vi "SetFlowRate.vi"(7 "Timeout (ms)":u32=2000, 8 "Error In":errorcluster, 10 "Flow Rate (mL/min)":dbl format="%.1f", 11 "Sierra M100 In":refnum<visa-resource-name>) -> (0 "Error Out":errorcluster, 2 "Set?":bool, 3 "Sierra M100 Out":refnum<visa-resource-name>)   [LabVIEW 2012, in "Sierra-M100.lvlib"]
doc: "This VI is sets the flow rate. Use this VI when unsure which of the other VIs to use for setting the flow rate setpoint."
uses:
  Sierra-M100.lvlib
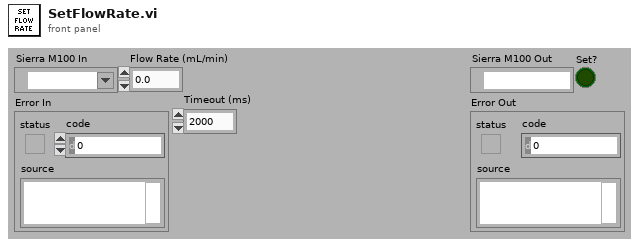
[diagram p1: front panel]
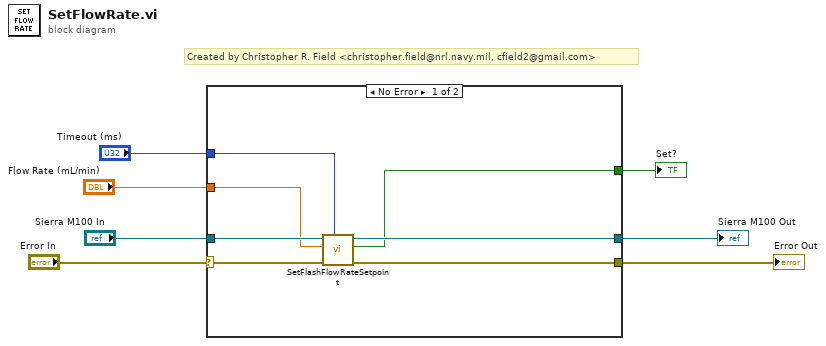
[diagram p0: block diagram]
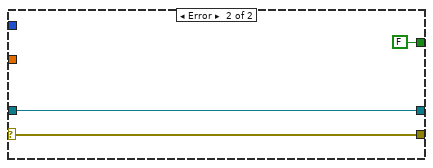
[diagram p2: hidden frame]
diagram:
  # "Created by Christopher R. Field <christopher.field@nrl.navy.mil, cfield2@gmail.com>"
  n1 = case shown="No Error" "Error In" {
    selector: "Error In" -> [w8 w16]
    tunnel: "Sierra M100 In" -> [w14 w17]
    tunnel: [w13 w17] -> w6
    tunnel: [w12 w16] -> w5
    tunnel: "Flow Rate (mL/min)" -> [w11 _]
    tunnel: "Timeout (ms)" -> [w10 _]
    tunnel: [w9 FALSE ("Set?")] -> w2
    frame No Error {
      n2 = call "SetFlashFlowRateSetpoint.vi"("Timeout (ms)"=w10, "Error In"=w8, "Setpoint (mL/min)"=w11, "Sierra M100 In"=w14) -> ("Error Out"=w12:errorcluster, "Set?"=w9:bool, "Sierra M100 Out"=w13:refnum<visa-resource-name>)  [unwired: 5 in]
    }
    frame Error {
    }
  }
  "Sierra M100 Out" <- w6
  "Error Out" <- w5
  "Set?" <- w2
